vi "Set Refnums.vi"   [LabVIEW 2014]
uses:
  Global Variables.vi
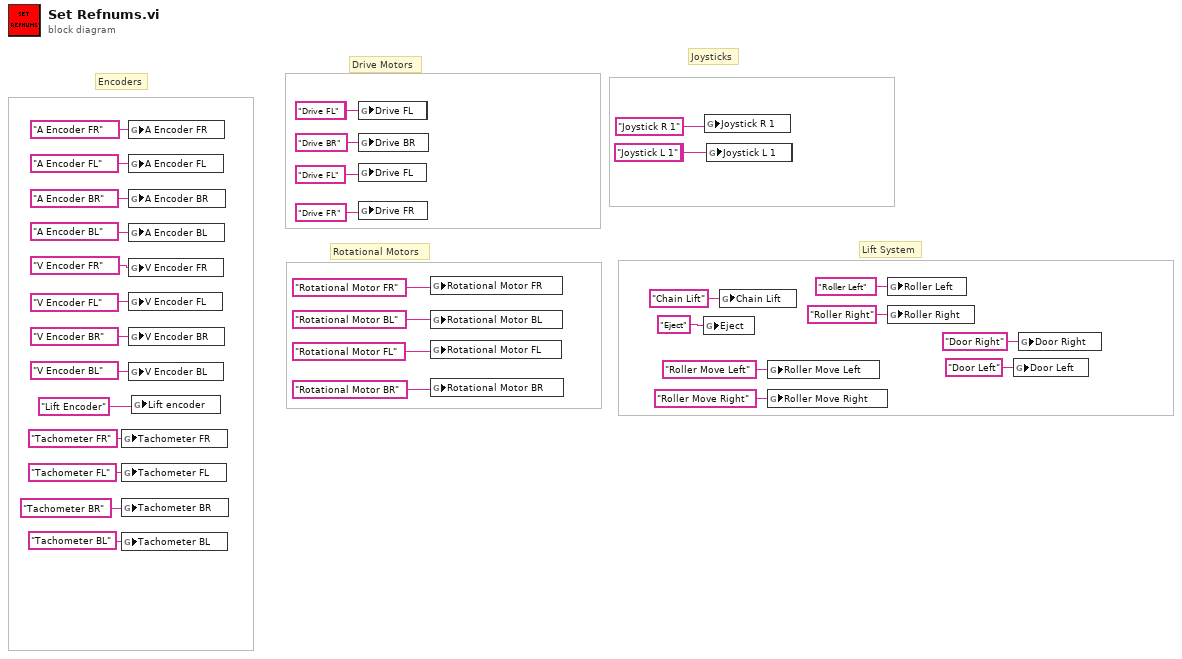
[diagram p0: block diagram]
diagram:
  # "Lift System"
  # "Rotational Motors"
  # "Encoders"
  # "Joysticks"
  # "Drive Motors"
  n1 = global write "Global Variables.vi" "Tachometer FR"("Tachometer FR") -> ()
  n2 = global write "Global Variables.vi" "Tachometer FL"("Tachometer FL") -> ()
  n3 = global write "Global Variables.vi" "Tachometer BR"("Tachometer BR") -> ()
  n4 = global write "Global Variables.vi" "Tachometer BL"("Tachometer BL") -> ()
  n5 = global write "Global Variables.vi" "A Encoder FR"("A Encoder FR") -> ()
  n6 = global write "Global Variables.vi" "A Encoder FL"("A Encoder FL") -> ()
  n7 = global write "Global Variables.vi" "A Encoder BR"("A Encoder BR") -> ()
  n8 = global write "Global Variables.vi" "A Encoder BL"("A Encoder BL") -> ()
  n9 = global write "Global Variables.vi" "V Encoder FR"("V Encoder FR") -> ()
  n10 = global write "Global Variables.vi" "V Encoder FL"("V Encoder FL") -> ()
  n11 = global write "Global Variables.vi" "V Encoder BR"("V Encoder BR") -> ()
  n12 = global write "Global Variables.vi" "V Encoder BL"("V Encoder BL") -> ()
  n13 = global write "Global Variables.vi" "Lift encoder"("Lift Encoder" ("Lift encoder")) -> ()
  n14 = global write "Global Variables.vi" "Drive BL"("Drive BL") -> ()
  n15 = global write "Global Variables.vi" "Drive FL"("Drive FL") -> ()
  n16 = global write "Global Variables.vi" "Drive FR"("Drive FR") -> ()
  n17 = global write "Global Variables.vi" "Drive BR"("Drive BR") -> ()
  n18 = global write "Global Variables.vi" "Drive FL"("Drive FL") -> ()
  n19 = global write "Global Variables.vi" "Drive FR"("Drive FR") -> ()
  n20 = global write "Global Variables.vi" "Rotational Motor FR"("Rotational Motor FR") -> ()
  n21 = global write "Global Variables.vi" "Rotational Motor BL"("Rotational Motor BL") -> ()
  n22 = global write "Global Variables.vi" "Rotational Motor FL"("Rotational Motor FL") -> ()
  n23 = global write "Global Variables.vi" "Rotational Motor BR"("Rotational Motor BR") -> ()
  n24 = global write "Global Variables.vi" "Eject"("Eject") -> ()
  n25 = global write "Global Variables.vi" "Joystick R 1"("Joystick R 1" ("Joystick R 1")) -> ()
  n26 = global write "Global Variables.vi" "Joystick L 1"("Joystick L 1" ("Joystick R 1")) -> ()
  n27 = global write "Global Variables.vi" "Joystick R 1"("Joystick R 1" ("Joystick R 1")) -> ()
  n28 = global write "Global Variables.vi" "Chain Lift"("Chain Lift") -> ()
  n29 = global write "Global Variables.vi" "Roller Move Left"("Roller Move Left") -> ()
  n30 = global write "Global Variables.vi" "Roller Move Right"("Roller Move Right") -> ()
  n31 = global write "Global Variables.vi" "Roller Left"("Roller Left") -> ()
  n32 = global write "Global Variables.vi" "Roller Right"("Roller Right") -> ()
  n33 = global write "Global Variables.vi" "Door Left"("Door Left") -> ()
  n34 = global write "Global Variables.vi" "Door Right"("Door Right") -> ()
